vi "play_audio.vi"(2 "Sound_name":u16(ring) items=["reach_out", "FR_yes", "FR_no", "EN_yes", "EN_no", "explo", "completed", "applause"]) -> (0 "error out":errorcluster)   [LabVIEW 2012]
uses:
  Global_var.vi
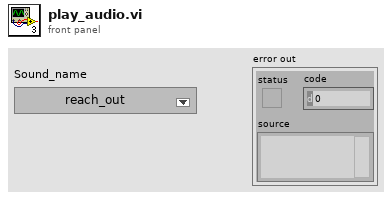
[diagram p1: front panel]
types:
  T1 = typedef "Sound Output Task ID.ctl" = u32
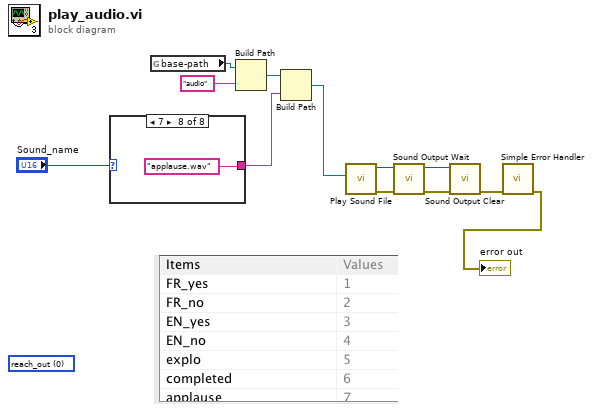
[diagram p0: block diagram]
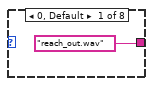
[diagram p2: hidden frame]
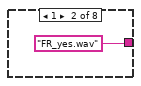
[diagram p3: hidden frame]
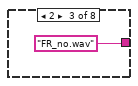
[diagram p4: hidden frame]
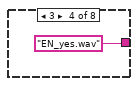
[diagram p5: hidden frame]
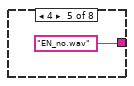
[diagram p6: hidden frame]
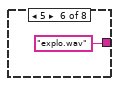
[diagram p7: hidden frame]
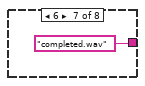
[diagram p8: hidden frame]
diagram:
  (unwired) u16 0 items=["reach_out", "FR_yes", "FR_no", "EN_yes", "EN_no", "explo", "completed", "applause"] ("Sound_name")
  n1 = case shown="7" "Sound_name" {
    tunnel: ["reach_out.wav" ("name or relative path") "FR_yes.wav" ("name or relative path") "FR_no.wav" ("name or relative path") "EN_yes.wav" ("name or relative path") "EN_no.wav" ("name or relative path") "explo.wav" ("name or relative path") "completed.wav" ("name or relative path") "applause.wav" ("name or relative path")] -> w5
    frame 0, Default {
    }
    frame 1 {
    }
    frame 2 {
    }
    frame 3 {
    }
    frame 4 {
    }
    frame 5 {
    }
    frame 6 {
    }
    frame 7 {
    }
  }
  n2 = global read "Global_var.vi" "base-path"() -> (w7:path)
  n3 = Build Path(base path=w7, name or relative path="audio") -> (appended path=w6:path)
  n4 = Build Path(base path=w6, name or relative path=w5) -> (appended path=w4:path)
  n5 = call <vilib>:"Play Sound File.vi"("path"=w4) -> ("error out"=w12:errorcluster, "task ID"=w11:T1)  [unwired: 9 in]
  n6 = call <vilib>:"Sound Output Wait.vi"("error in (no error)"=w12, "task ID"=w11) -> ("error out"=w2:errorcluster, "task ID out"=w3:T1)  [unwired: 8 in]
  n7 = call <vilib>:"Sound Output Clear.vi"("error in (no error)"=w2, "task ID"=w3) -> ("error out"=w9:errorcluster)  [unwired: 9 in]
  n8 = call <vilib>:"Simple Error Handler.vi"("error in (no error)"=w9) -> ("error out"=→"error out":errorcluster)  [unwired: 4 in, 4 out]
